vi "APS set trigger table.vi"(7 "ArraySize":i32, 8 "error in (no error)":errorcluster caption="错误输入（无错误）", 9 "DataArr":i32, 10 "TCmpCh":i32, 11 "Board_ID":i32) -> (0 "error out":errorcluster caption="错误输出", 1 "DataArr out":i32, 3 "function return":i32)   [LabVIEW 2011, in "APS168.lvlib"]
doc: "I32 FNTYPE APS_set_trigger_table( I32 Board_ID, I32 TCmpCh, I32 *DataArr, I32 ArraySize );"
uses:
  APS168.lvlib
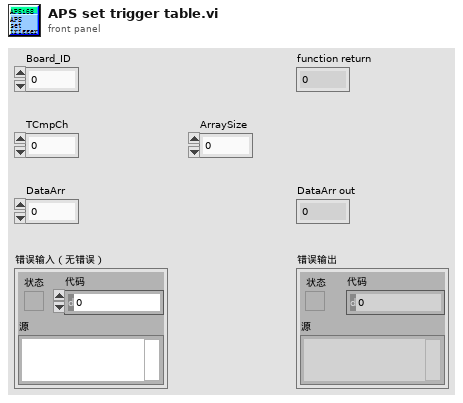
[diagram p1: front panel]
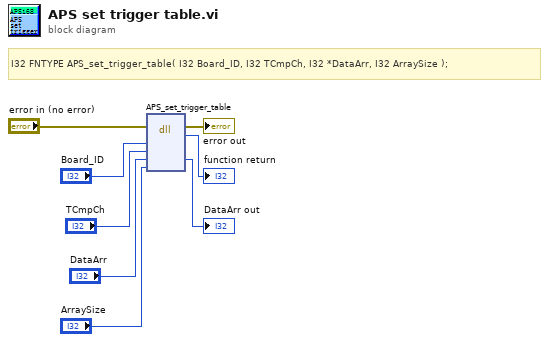
[diagram p0: block diagram]
diagram:
  # "I32 FNTYPE APS_set_trigger_table( I32 Board_ID, I32 TCmpCh, I32 *DataArr, I32 ArraySize );"
  n1 = dll-call lib="PTH1Labs E软件ADLINK 204CAPS_1_7_1_LIB line 连续运动204APS168.*" fn="APS_set_trigger_table"(error in="error in (no error)", "Board_ID"="Board_ID", "TCmpCh"="TCmpCh", "DataArr"="DataArr", "ArraySize"="ArraySize") -> (error out=→"error out":errorcluster, →"function return":i32, "DataArr"=→"DataArr out":i32)  [unwired: 5 in, 1 out]
